vi "2_static_friction_main.vi"() -> ()   [LabVIEW 2019]
uses:
  helper_vis/TypeDef_Static_Friction.ctl
  helper_vis/TypeDef_Current_Setting.ctl
  Shared VIs/ENPID/PID_Settings.ctl
  Shared VIs/ENPID/Gains.ctl
  Shared VIs/ENPID/NonLinearGainParams.ctl
  Shared VIs/ENPID/NonLinearGain.ctl
  Shared VIs/ENPID/DPartVariable.ctl
  Shared VIs/ENPID/VelocityEstimate.ctl
  Shared VIs/ENPID/OutputRange.ctl
  Shared VIs/TypeDef_TDMS_States.ctl
  <vilib>/myRIO/Common/Instrument Driver Framework/myRIO v1.0/Encoder/typedefs/Encoder Signal Mode.ctl
  Shared VIs/ModelSpecific/ETHMikeModel.ctl
  Shared VIs/ModelSpecific/ReadOnlyGlobalActions.ctl
  <vilib>/myRIO/Instrument Drivers/Onboard IO/AI/typedefs/AI Reference.ctl
  <vilib>/myRIO/Common/Instrument Driver Framework/Utilities/typedefs/myRIO Generic Hardware Reference.ctl
  <vilib>/myRIO/Common/Instrument Driver Framework/Utilities/typedefs/Hardware Version Enum.ctl
  <vilib>/myRIO/Common/Instrument Driver Framework/Utilities/typedefs/myRIO v1.0 Reference.ctl
  <vilib>/myRIO/Common/Instrument Driver Framework/Utilities/typedefs/Generic FPGA Reference.ctl
  <vilib>/myRIO/Common/Instrument Driver Framework/myRIO v1.0/AI/typedefs/AI Channels List.ctl
  <vilib>/myRIO/Common/Instrument Driver Framework/myRIO v1.0/AI/typedefs/AI Channels Enum.ctl
  <vilib>/myRIO/Common/Instrument Driver Framework/Utilities/typedefs/Analog Scaling Constants List.ctl
  <vilib>/myRIO/Common/Instrument Driver Framework/Utilities/typedefs/Analog Scaling Constants.ctl
  <vilib>/userDefined/High Color/nirio_resource_hc.ctl
  <vilib>/myRIO/Instrument Drivers/Onboard IO/AO/typedefs/AO Reference.ctl
  <vilib>/myRIO/Common/Instrument Driver Framework/myRIO v1.0/AO/typedefs/AO Channels List.ctl
  <vilib>/myRIO/Common/Instrument Driver Framework/myRIO v1.0/AO/typedefs/AO Channels Enum.ctl
  <vilib>/Platform/TimedLoop/XDataNode/timing_clust.ctl
  <vilib>/Platform/TimedLoop/XDataNode/nitl_modes.ctl
  <vilib>/Platform/TimedLoop/XDataNode/wakeup.ctl
  <vilib>/Analysis/3filter.llb/Filter Passband Type.ctl
  <vilib>/myRIO/Common/Instrument Driver Framework/myRIO v1.0/AI/vis/myRIO v1.1 Open AI.vi
  <vilib>/myRIO/Common/Instrument Driver Framework/myRIO v1.0/AO/vis/myRIO v1.1 Open AO.vi
  <vilib>/myRIO/Common/Instrument Driver Framework/Utilities/vis/Validate Channels.vi
  <vilib>/myRIO/Common/Instrument Driver Framework/myRIO v1.0/AI/vis/myRIO v1.0 Reserve AI.vi
  <vilib>/myRIO/Common/Instrument Driver Framework/myRIO v1.0/AO/vis/myRIO v1.0 Reserve AO.vi
  <vilib>/myRIO/Common/Instrument Driver Framework/myRIO v1.0/AI/vis/myRIO v1.0 Close AI.vi
  <vilib>/myRIO/Common/Instrument Driver Framework/myRIO v1.0/Encoder/vis/myRIO v1.0 Close Encoder.vi
  <vilib>/myRIO/Common/Instrument Driver Framework/myRIO v1.0/AO/vis/myRIO v1.0 Close AO.vi
  <vilib>/myRIO/Common/Instrument Driver Framework/myRIO v1.0/AI/vis/myRIO v1.0 Build MUX Configuration AI.vi
  <vilib>/myRIO/Common/Instrument Driver Framework/myRIO v1.0/Resource Manager/vis/myRIO v1.0 Reserve Channel List.vi
  <vilib>/myRIO/Common/Instrument Driver Framework/myRIO v1.0/AO/vis/myRIO v1.0 Build MUX Configuration AO.vi
  <vilib>/myRIO/Common/Instrument Driver Framework/myRIO v1.0/AI/vis/myRIO v1.0 Unreserve AI.vi
  <vilib>/myRIO/Common/Instrument Driver Framework/myRIO v1.0/Encoder/vis/myRIO v1.0 Unreserve Encoder.vi
  <vilib>/myRIO/Common/Instrument Driver Framework/myRIO v1.0/AO/vis/myRIO v1.0 Unreserve AO.vi
  <vilib>/myRIO/Common/Instrument Driver Framework/myRIO v1.0/Resource Manager/vis/myRIO v1.0 Reserve Channel.vi
  <vilib>/myRIO/Common/Instrument Driver Framework/myRIO v1.0/Resource Manager/vis/myRIO v1.0 Unreserve Channel.vi
  <vilib>/myRIO/Common/Instrument Driver Framework/myRIO v1.0/Resource Manager/vis/myRIO v1.0 Unreserve Channel List.vi
  <vilib>/myRIO/Common/Instrument Driver Framework/myRIO v1.0/Encoder/vis/myRIO v1.0 Build MUX Configuration Encoder.vi
  <vilib>/myRIO/Common/Instrument Driver Framework/myRIO v1.0/Resource Manager/vis/myRIO v1.0 Build Mutex Name.vi
  <vilib>/myRIO/Common/Instrument Driver Framework/myRIO v1.0/Resource Manager/vis/myRIO v1.0 Create Configuration List.vi
  <vilib>/Utility/VariantDataType/GetNumericInfo.vi
  <vilib>/Utility/error.llb/Error Cluster From Error Code.vi
  <vilib>/myRIO/Common/Instrument Driver Framework/myRIO v1.0/myRIO v1.1 Open.vi
  <vilib>/myRIO/Common/Instrument Driver Framework/myRIO v1.0/AO/vis/myRIO v1.0 Get Scaling Constants AO.vi
  <vilib>/myRIO/Common/Instrument Driver Framework/Utilities/vis/IO Manager.vi
  <vilib>/myRIO/Common/Instrument Driver Framework/Utilities/vis/Configuration Manager.vi
  <vilib>/myRIO/Common/Instrument Driver Framework/myRIO v1.0/myRIO v1.0 Close.vi
  <vilib>/myRIO/Common/Instrument Driver Framework/myRIO v1.0/AO/vis/myRIO v1.0 Write AO.vi
  <vilib>/myRIO/Common/Instrument Driver Framework/myRIO v1.0/AI/vis/myRIO v1.0 Get Scaling Constants AI.vi
  <vilib>/myRIO/Common/Instrument Driver Framework/myRIO v1.0/Encoder/vis/myRIO v1.0 Read Encoder.vi
  <vilib>/myRIO/Common/Instrument Driver Framework/myRIO v1.0/AI/vis/myRIO v1.0 Read AI.vi
  <vilib>/myRIO/Common/Instrument Driver Framework/myRIO v1.0/Encoder/vis/myRIO v1.0 Enable Encoder.vi
  <vilib>/myRIO/Common/Instrument Driver Framework/myRIO v1.0/Encoder/vis/myRIO v1.0 Shutdown Encoder.vi
  <vilib>/myRIO/Common/Instrument Driver Framework/myRIO v1.0/Resource Manager/vis/myRIO v1.0 Configure IO.vi
  <vilib>/myRIO/Instrument Drivers/Onboard IO/AO/vis/myRIO AO Open.xnode
  <vilib>/myRIO/Instrument Drivers/Onboard IO/AI/vis/myRIO AI Open.xnode
  <vilib>/Platform/TimedLoop/XDataNode/XDataNode.xnode
  <vilib>/myRIO/Instrument Drivers/Onboard IO/AO/AO.lvlib
  <vilib>/myRIO/Instrument Drivers/Onboard IO/Encoder/Encoder.lvlib
  <vilib>/myRIO/Instrument Drivers/Onboard IO/AI/AI.lvlib
  <vilib>/addons/control/pid/NI_PID_pid.lvlib
  <vilib>/Analysis/NI_AALBase.lvlib
  <vilib>/ptbypt/NI_PtbyPt.lvlib
  <vilib>/Platform/TimedLoop/XDataNode/XDNodeRunTimeDep.lvlib
panel:
  in  "TDMS Storage File Input":string
  out "TDMS States":T1
  in  "PID Settings":T2={"Gains"={"K(e)"=0.0, "Kp"=0.800000011920929, "Ki"=0.0, "Kd"=0.003000000026077032}, "Non-linear gain"={"Non-linear gain P"=enum."off", "Non-linear gain I"=enum."off", "Non-linear gain D"=enum."off"}, "D-Part variable"=enum."process variable", "Velocity estimate dy/dt"=enum."external", "Anti reset windup"=TRUE, "I-Part error band"=inf, "Output range"={"output high"=0.0, "output low"=0.0}}
  in  "Save data?":bool
  out "Final Current Setpoint":dbl
  out "Boolean: Apply Current":bool
  out "Boolean: Move":bool
  out "Position Difference [deg]":dbl
  in  "move":bool
  out "Profile Complete?":bool
  in  "Current Direction [+/-]":T9
  out "Velocity [deg/s]":dbl
  in  "Actions":T10
  out "Current Setpoint [A]":dbl
  out "Position [deg] Chart":dbl(graph)
  out "Current [A] Chart":dbl(graph)
  out "Position [deg]":dbl
  in  "stop":bool
  out "Current [A]":dbl
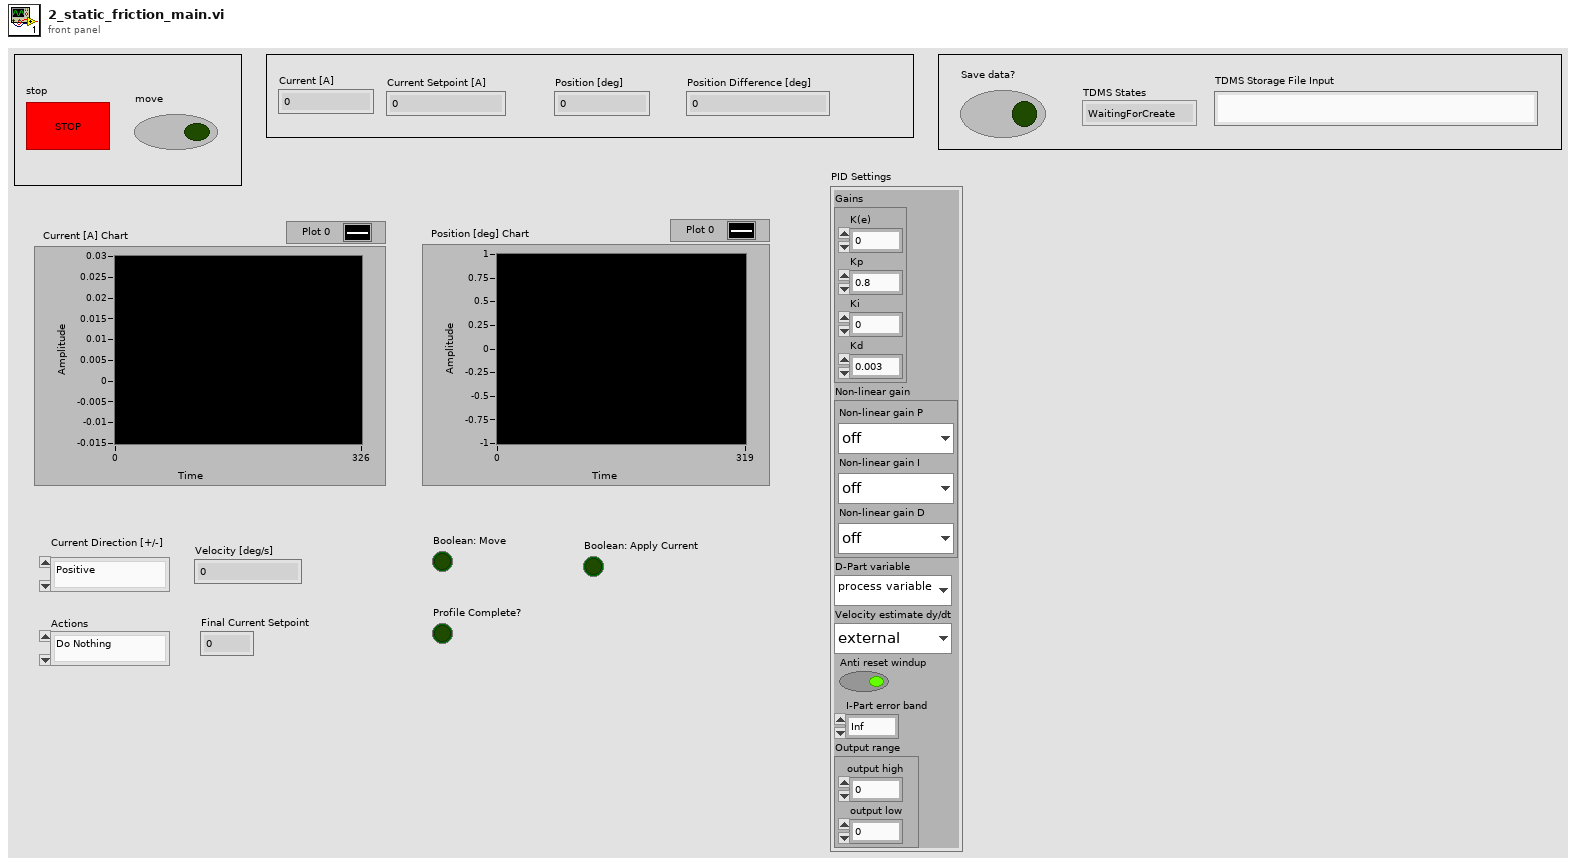
[diagram p1: front panel]
types:
  T1 = typedef "TypeDef_TDMS_States.ctl" = enum16{"WaitingForCreate", "Create", "Buffering", "Flushing", "Write", "Close"}
  T2 = typedef "PID_Settings.ctl" = cluster{"Gains":T3, "Non-linear gain":T4, "D-Part variable":T6, "Velocity estimate dy/dt":T7, "Anti reset windup":bool, "I-Part error band":dbl, "Output range":T8}
  T3 = typedef "Gains.ctl" = cluster{"K(e)":dbl, "Kp":dbl, "Ki":dbl, "Kd":dbl}
  T4 = typedef "NonLinearGainParams.ctl" = cluster{"Non-linear gain P":T5, "Non-linear gain I":T5, "Non-linear gain D":T5}
  T5 = typedef "NonLinearGain.ctl" = enum16{"exponential", "quadratic", "off"}
  T6 = typedef "DPartVariable.ctl" = enum16{"error", "process variable"}
  T7 = typedef "VelocityEstimate.ctl" = enum16{"derivative", "external"}
  T8 = typedef "OutputRange.ctl" = cluster{"output high":dbl, "output low":dbl}
  T9 = typedef "TypeDef_Current_Setting.ctl" = enum16{"Positive", "Negative"}
  T10 = typedef "TypeDef_Static_Friction.ctl" = enum16{"Do Nothing", "Move", "Wait", "Apply Current"}
  T11 = typedef "nirio_resource_hc.ctl" = tag
  T12 = typedef "Hardware Version Enum.ctl" = enum16{"Unknown", "myRIO-1900", "myRIO-1950", "roboRIO", "NI ELVIS RIO CM", "ELVIS III"}
  T13 = enum16{"open", "open or create", "create or replace", "create", "open (read-only)"}
  T14 = typedef "XDNodeRunTimeDep.lvlib/timing_clust.ctl" = cluster{"Expected End [f-1]":u64, "Actual End [f-1]":u64, "Finished Late? [f-1]":bool, "Expected End [i-1]":u64, "Actual End [i-1]":u64, "Finished Late? [i-1]":bool, "Expected Start [i]":u64, "Actual Start [i]":u64, "Expected Start [f]":u64, "Actual Start [f]":u64, "Source Name":string, "Structure Name":string, "Period":i64, "Deadline":i64, "Offset":i64, "Start":i64, "Priority":i32, "Timeout":i32, "Mode":T15, "Wakeup Reason":T16, "Error":errorcluster, "Source Type":string, "Secondary Source Type":string, "Global End Time":u64, "Global Start Time":u64, "Frame Duration":u64, "Iteration Duration":u64, "Assigned CPU":i32, "I/O Scan Engine Mode":u32}
  T15 = typedef "XDNodeRunTimeDep.lvlib/nitl_modes.ctl" = enum32{"No Change", "Process missed periods, maintain original phase", "Discard missed periods, maintain original phase", "Process missed periods, ignore original phase", "Discard missed periods, ignore original phase"}
  T16 = typedef "XDNodeRunTimeDep.lvlib/wakeup.ctl" = enum32{"Normal", "Aborted", "Asynchronous wakeup", "Timing source error", "Timed loop error", "Timeout"}
  T17 = typedef "NI_AALBase.lvlib/Filter Passband Type.ctl" = enum32{"Lowpass", "Highpass", "Bandpass", "Bandstop"}
  T18 = typedef "ReadOnlyGlobalActions.ctl" = enum16{"Initialize", "Read", "Write"}
  T19 = typedef "ETHMikeModel.ctl" = enum16{"ETH Mike #1", "ETH Mike #2", "ETH Mike #3", "ETH Mike #4", "ETH MIKE #5"}
  T20 = typedef "Encoder Signal Mode.ctl" = enum16{"Quadrature phase signal", "Step and direction signal"}
  T21 = typedef "AO.lvlib/AO Reference.ctl" = cluster{"myRIO Reference":T22, "AO Channel List":T25, "AO Scaling Constant List":T27}
  T22 = typedef "myRIO Generic Hardware Reference.ctl" = cluster{"myRIO Model":T12, "myRIO Hardware Reference":T23}
  T23 = typedef "myRIO v1.0 Reference.ctl" = cluster{"Generic FPGA Reference":T24, "Allow multiple opens":bool}
  T24 = typedef "Generic FPGA Reference.ctl" = refnum<k20>
  T25 = typedef "AO Channels List.ctl" = T26[]
  T26 = typedef "AO Channels Enum.ctl" = enum16{"Not Connected", "AudioOut/Left", "AudioOut/Right", "C/AO0", "C/AO1", "A/AO0", "A/AO1", "B/AO0", "B/AO1"}
  T27 = typedef "Analog Scaling Constants List.ctl" = T28[]
  T28 = typedef "Analog Scaling Constants.ctl" = cluster{"LSB Weight (Volts)":dbl, "Offset (Volts)":dbl, "Signed?":bool}
  T29 = typedef "Encoder.lvlib/Encoder Reference.ctl" = cluster{"myRIO Reference":T22, "Encoder Channels Enum":T30}
  T30 = typedef "Encoder Channels Enum.ctl" = enum16{"Not Connected", "C/ENC0", "C/ENC1", "A/ENC", "A/ENC0", "A/ENC1", "A/ENC2", "A/ENC3", "A/ENC4", "A/ENC5", "A/ENC6", "A/ENC7", "A/ENC8", "A/ENC9", "B/ENC", "B/ENC0", "B/ENC1", "B/ENC2", "B/ENC3", "B/ENC4", "B/ENC5", "B/ENC6", "B/ENC7", "B/ENC8", "B/ENC9", "DIO/ENC0", "DIO/ENC1", "DIO/ENC2", "DIO/ENC3", "DIO/ENC4"}
  T31 = typedef "AI.lvlib/AI Reference.ctl" = cluster{"myRIO Reference":T22, "AI Channels List":T32, "AI Scaling Constants List":T27}
  T32 = typedef "AI Channels List.ctl" = T33[]
  T33 = typedef "AI Channels Enum.ctl" = enum16{"Not Connected", "AudioIn/Left", "AudioIn/Right", "C/AI0", "C/AI1", "A/AI0", "A/AI1", "A/AI2", "A/AI3", "A/AI4", "A/AI5", "A/AI6", "A/AI7", "B/AI0", "B/AI1", "B/AI2", "B/AI3", "B/AI4", "B/AI5", "B/AI6", "B/AI7", "AI/AI0", "AI/AI1", "AI/AI2", "AI/AI3", "A/AI0 (DIFF)", "A/AI1 (DIFF)", "A/AI2 (DIFF)", "A/AI3 (DIFF)", "B/AI0 (DIFF)", "B/AI1 (DIFF)", "B/AI2 (DIFF)", "B/AI3 (DIFF)"}
  T34 = typedef "TypeDefTachometerParam.ctl" = cluster{"Offset [V]":dbl, "Gain [deg/sV]":dbl}
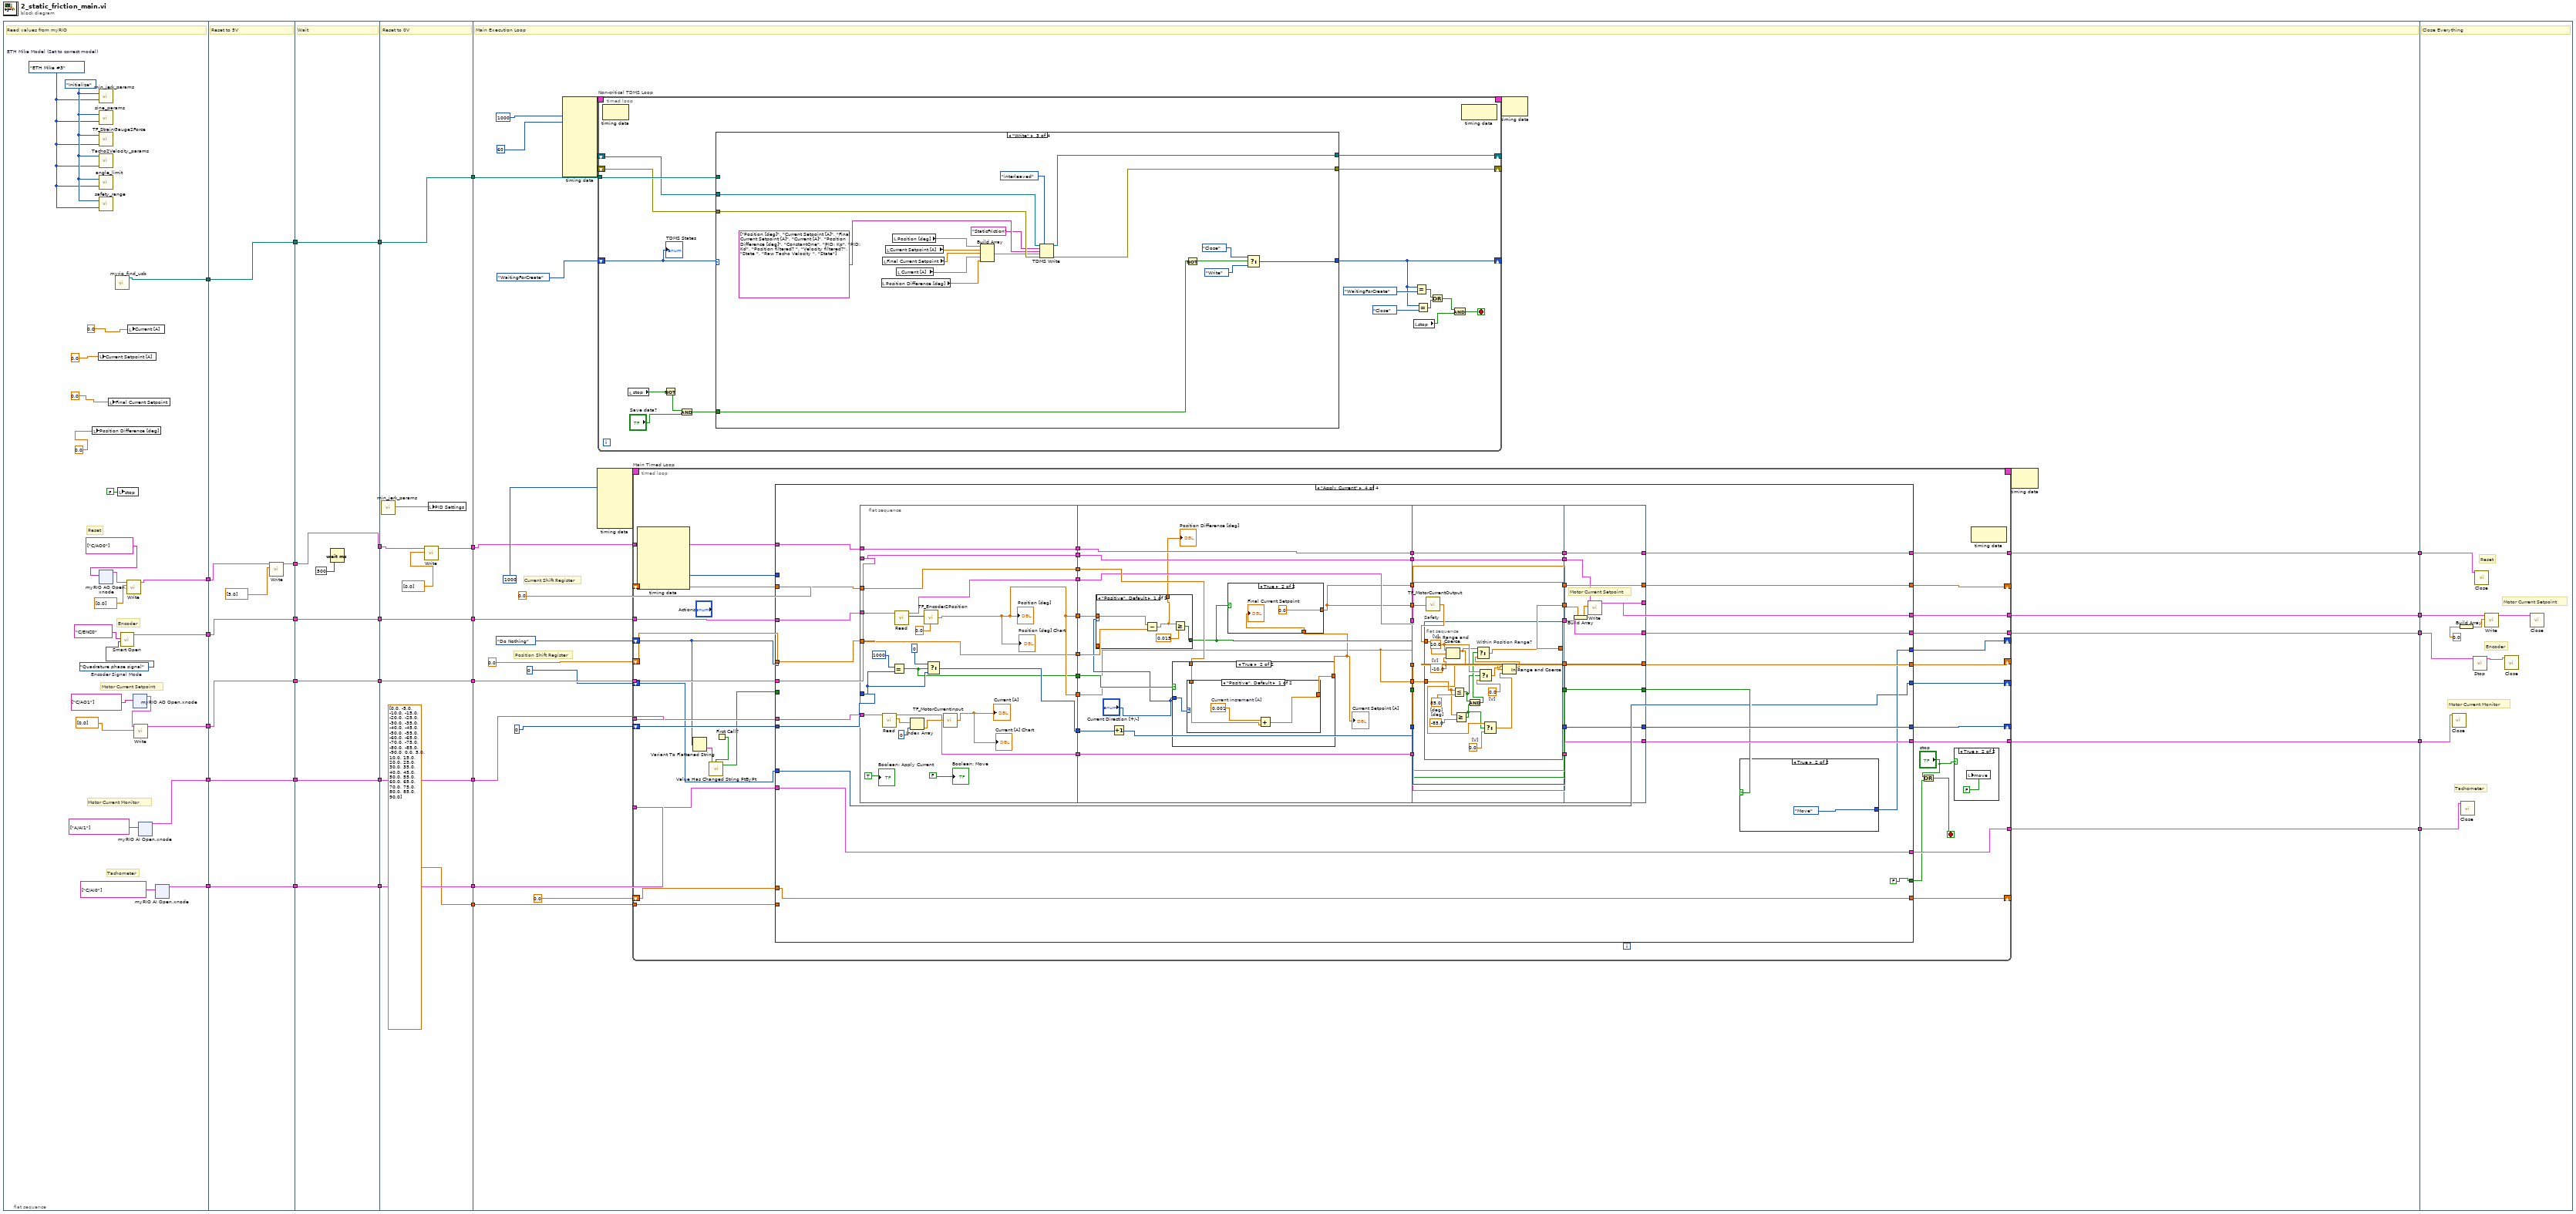
[diagram p0: block diagram]
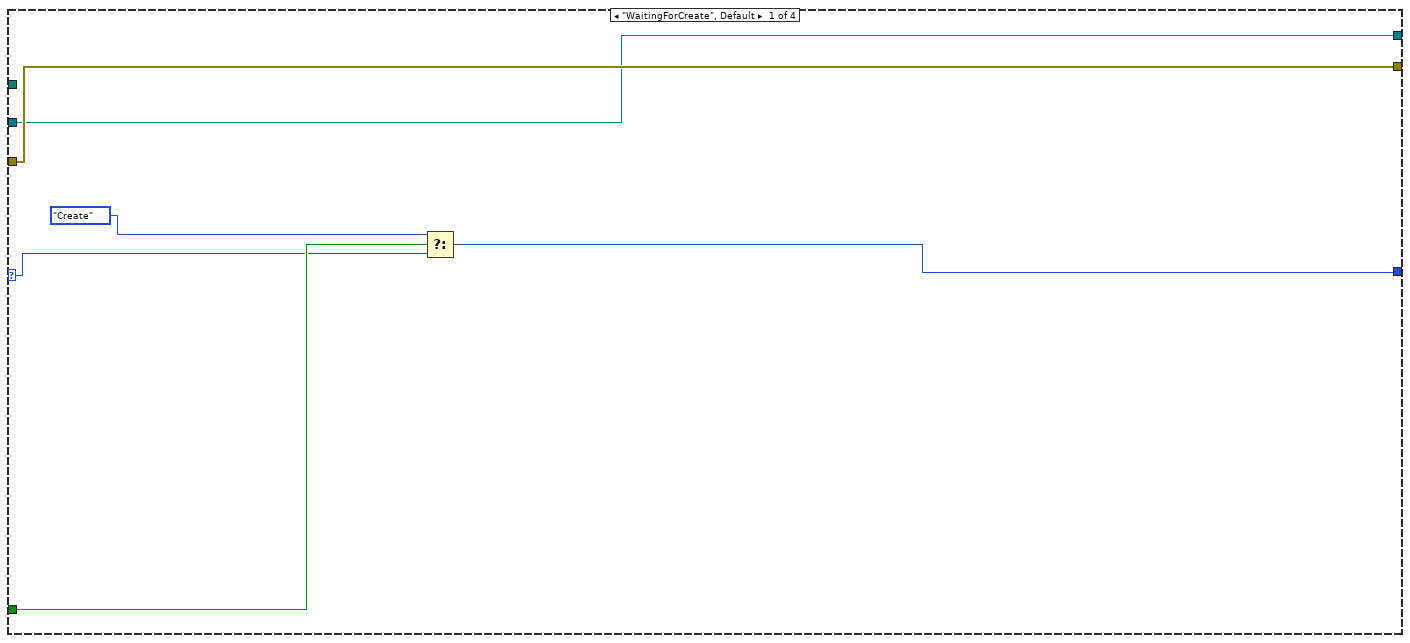
[diagram p2: hidden frame]
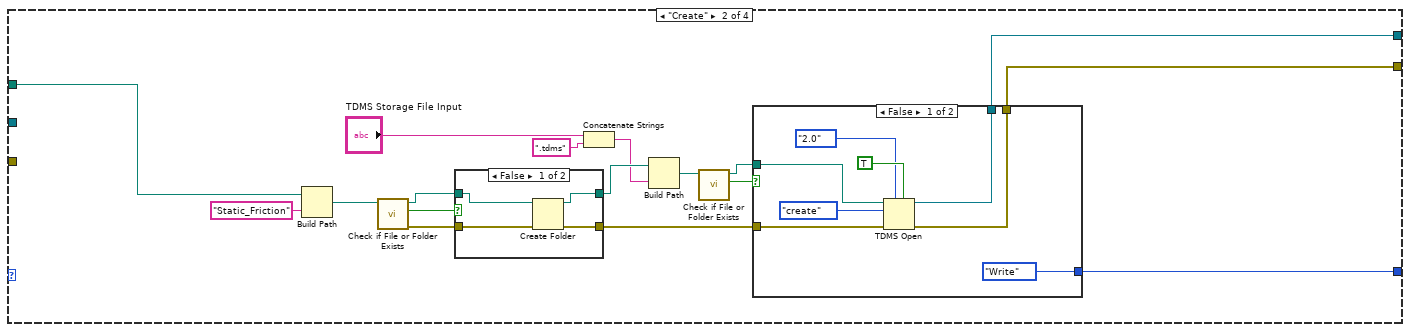
[diagram p3: hidden frame]
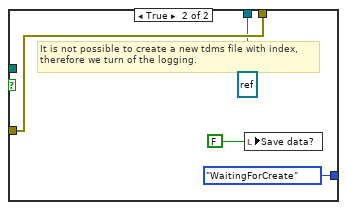
[diagram p4: hidden frame]
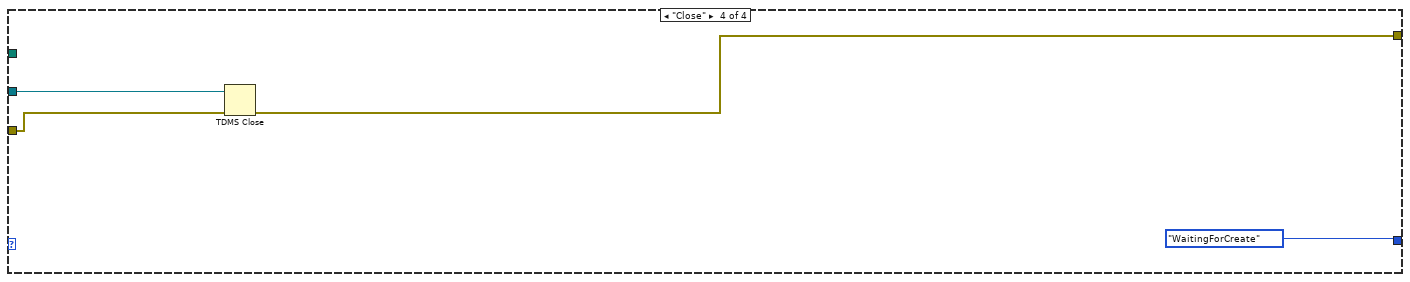
[diagram p6: hidden frame]
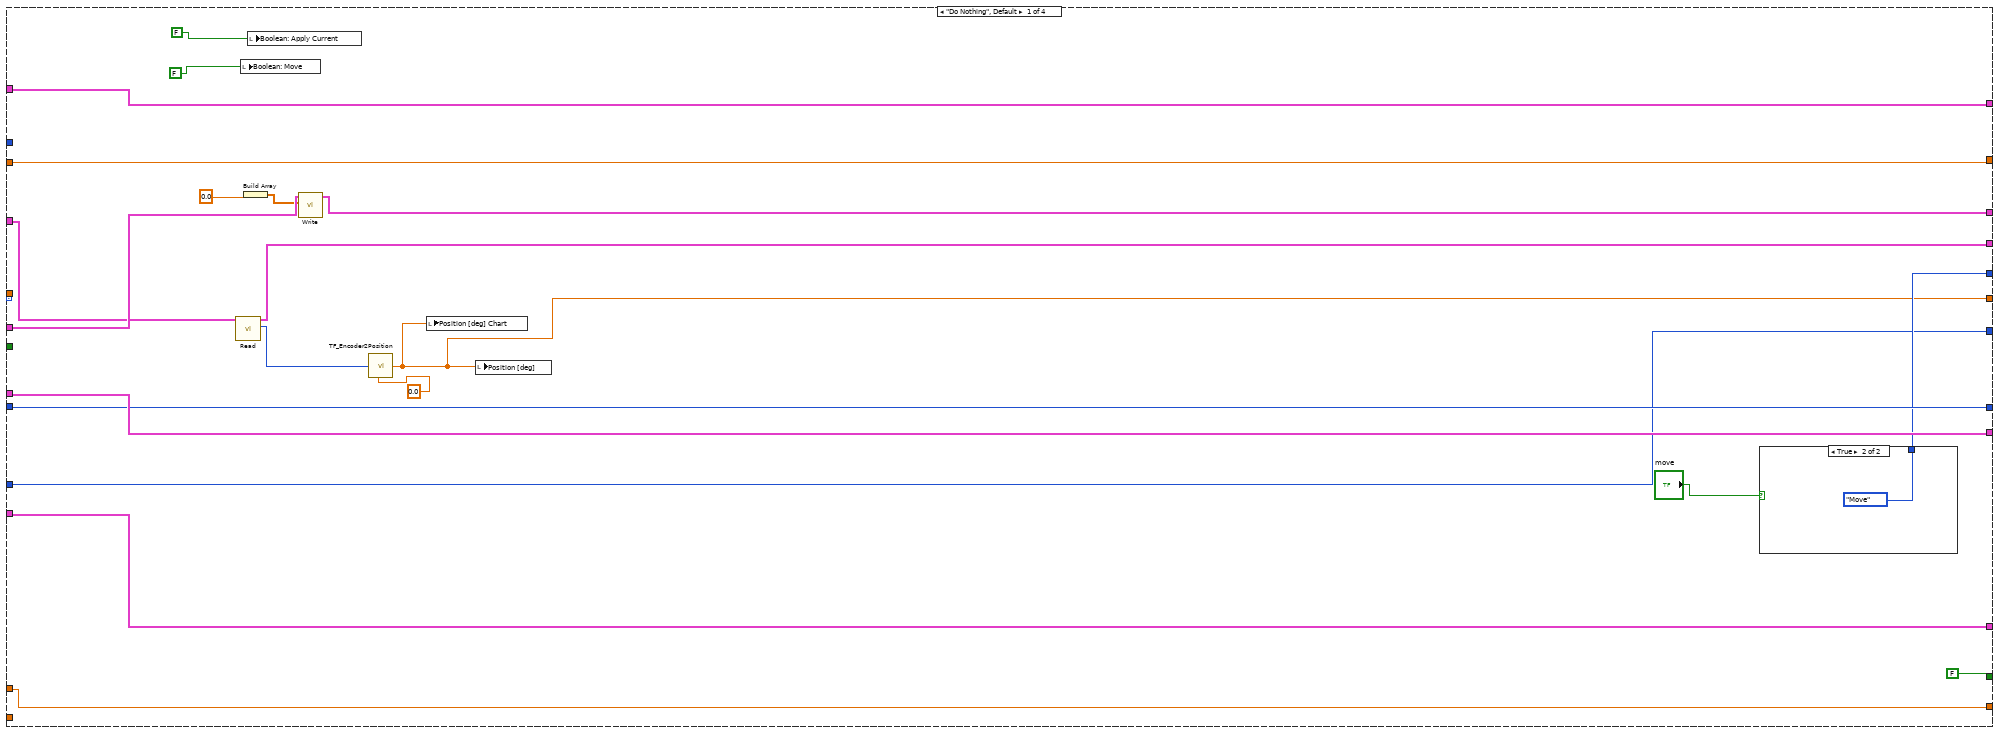
[diagram p8: hidden frame]
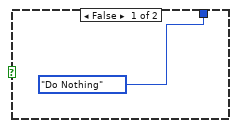
[diagram p9: hidden frame]
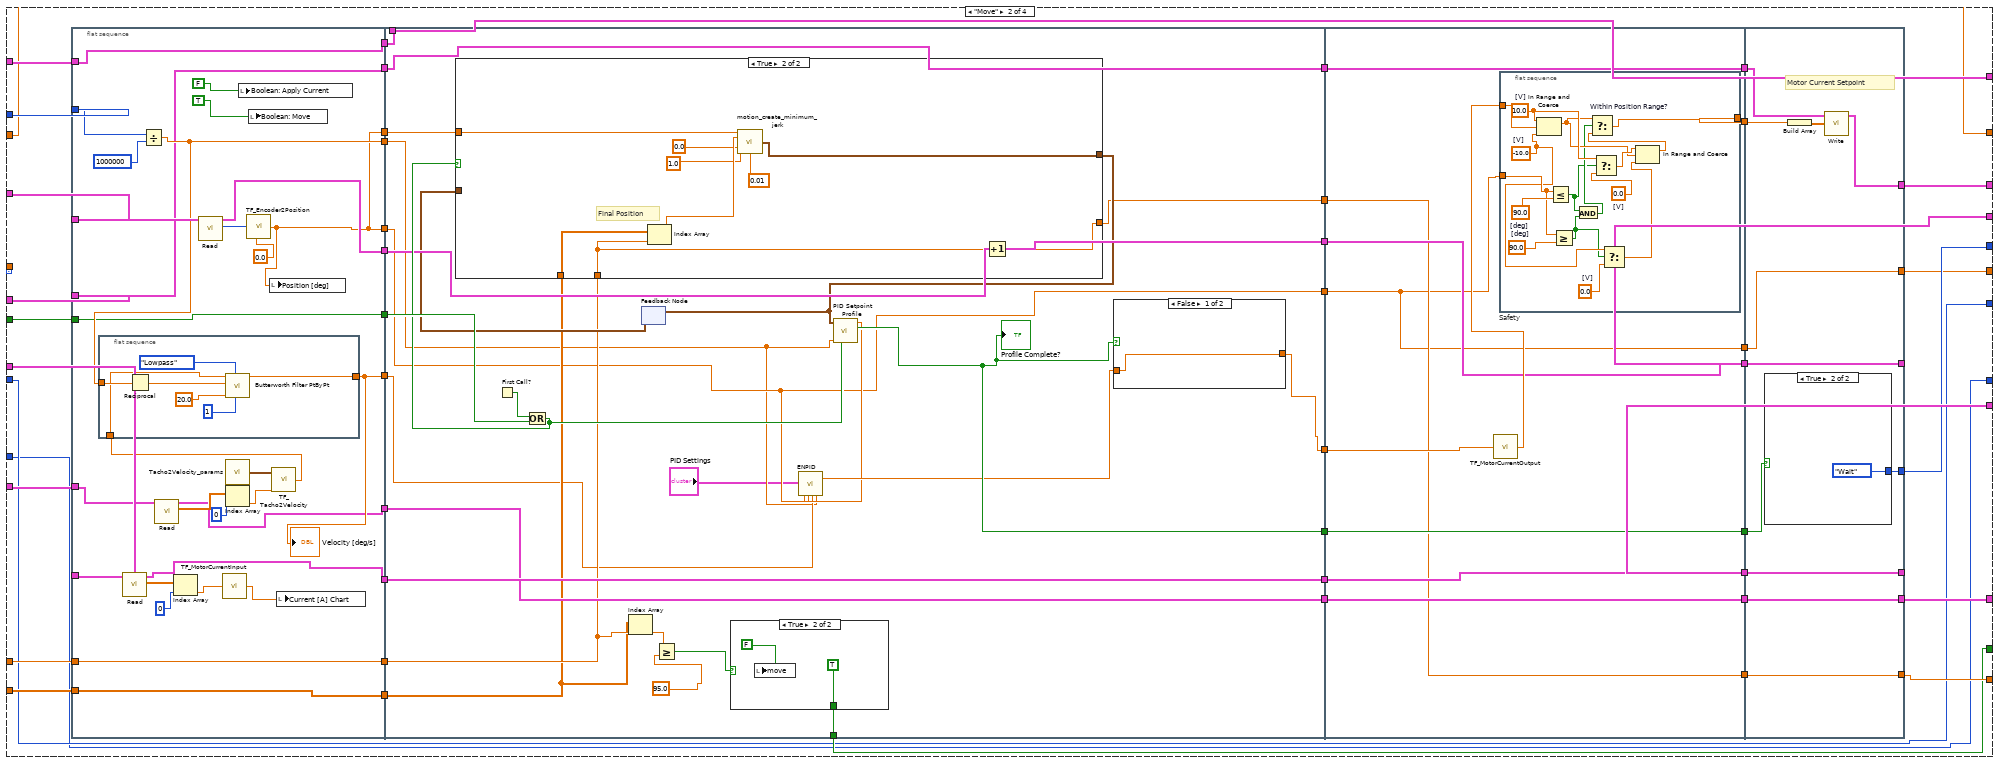
[diagram p10: hidden frame]
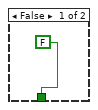
[diagram p11: hidden frame]
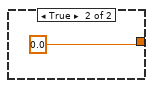
[diagram p12: hidden frame]
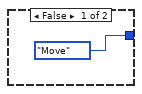
[diagram p14: hidden frame]
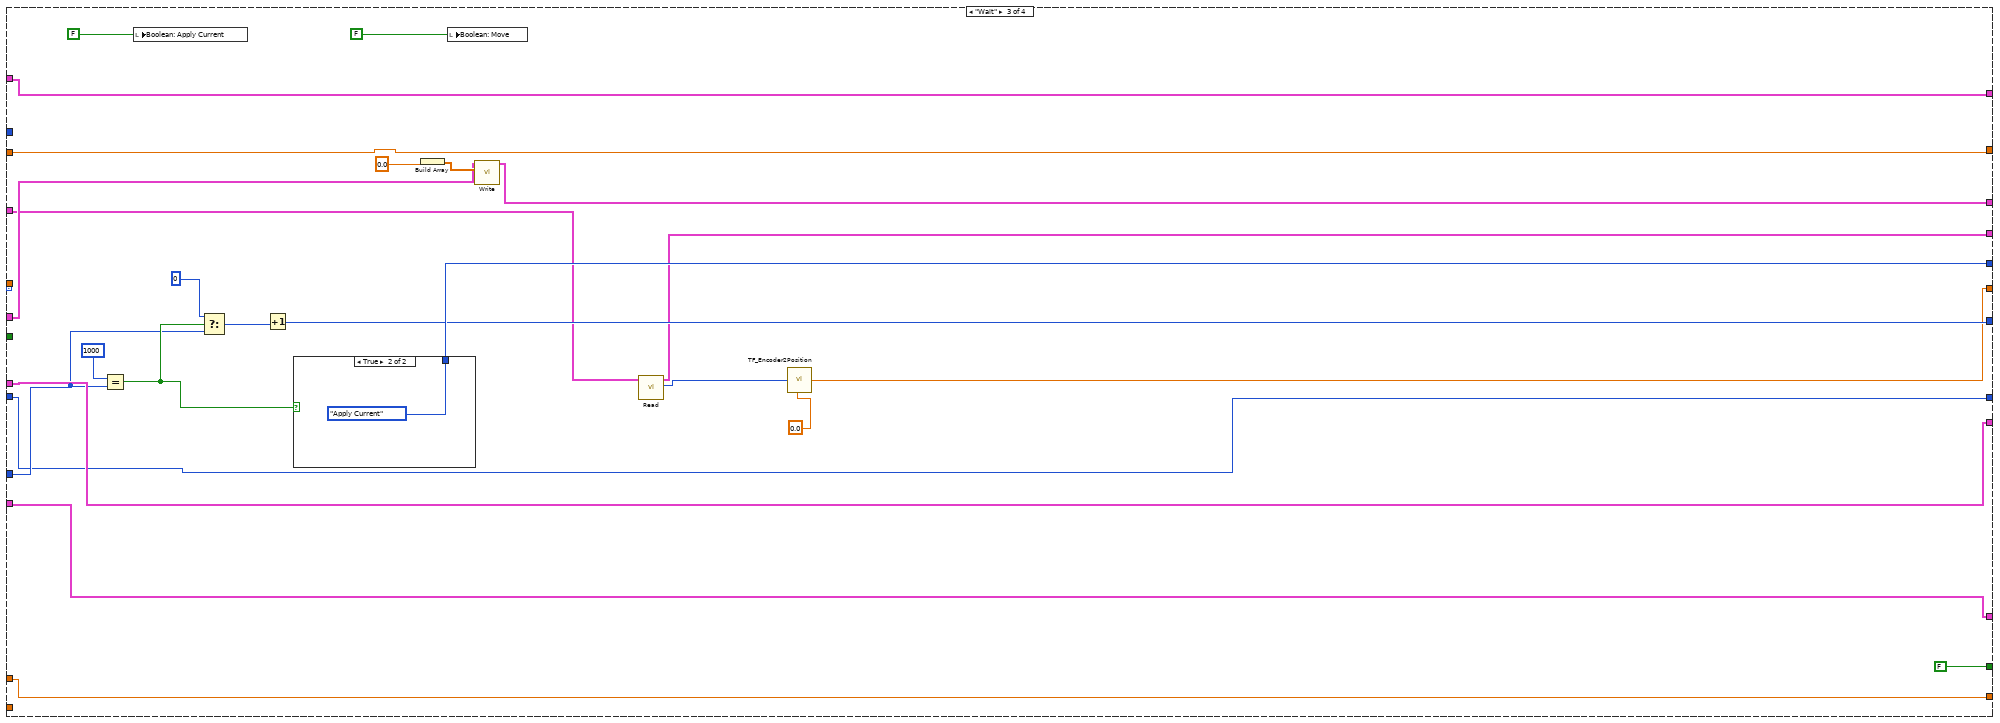
[diagram p15: hidden frame]
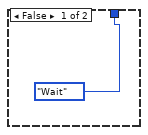
[diagram p16: hidden frame]
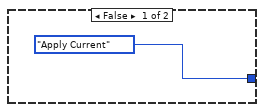
[diagram p17: hidden frame]
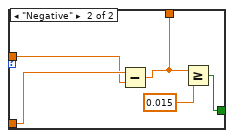
[diagram p18: hidden frame]
diagram:
  n1 = flat-sequence {
    tunnel: [w50] -> w30
    tunnel: [w47] -> w26
    tunnel: [w43] -> w25
    tunnel: [w41] -> w24
    tunnel: [w39] -> w7
    tunnel: [w38] -> w1
    tunnel: w30 -> [w132]
    tunnel: [w131] -> w28
    tunnel: w26 -> [w130]
    tunnel: w25 -> [w129]
    tunnel: w24 -> [w128]
    tunnel: [w130] -> w21
    tunnel: [w129] -> w18
    tunnel: [w128] -> w15
    tunnel: [w127] -> w8
    tunnel: w7 -> [w127]
    tunnel: [w126] -> w2
    tunnel: w1 -> [w126]
    tunnel: [w139] -> w29
    tunnel: w28 -> [w139]
    tunnel: [w138] -> w22
    tunnel: w21 -> [w138]
    tunnel: [w137] -> w19
    tunnel: w18 -> [w137]
    tunnel: [w136] -> w16
    tunnel: w15 -> [w136]
    tunnel: [w135] -> w9
    tunnel: w8 -> [w135]
    tunnel: [w134] -> w3
    tunnel: w2 -> [w134]
    tunnel: w29 -> [w149]
    tunnel: [w148] -> w27
    tunnel: [w147] -> w23
    tunnel: w22 -> [w147]
    tunnel: [w146] -> w20
    tunnel: w19 -> [w146]
    tunnel: [w145] -> w17
    tunnel: w16 -> [w145]
    tunnel: [w144] -> w10
    tunnel: w9 -> [w144]
    tunnel: [dbl[] [0.0, -5.0, -10.0, -15.0, -20.0, -25.0, -30.0, -35.0, -40.0, -45.0, -50.0, -55.0, -60.0, -65.0, -70.0, -75.0, -80.0, -85.0, -90.0, 0.0, 5.0, 10.0, 15.0, 20.0, 25.0, 30.0, 35.0, 40.0, 45.0, 50.0, 55.0, 60.0, 65.0, 70.0, 75.0, 80.0, 85.0, 90.0]] -> w5
    tunnel: [w142] -> w4
    tunnel: w3 -> [w142]
    tunnel: w27 -> [w169]
    tunnel: w23 -> [w173]
    tunnel: w20 -> [w172]
    tunnel: w17 -> [w163]
    tunnel: [w168] -> w14
    tunnel: [w167] -> w13
    tunnel: [w166] -> w12
    tunnel: [w165] -> w11
    tunnel: w10 -> [w164]
    tunnel: [w162] -> w6
    tunnel: w5 -> [w160]
    tunnel: w4 -> [w152]
    tunnel: w14 -> [w678]
    tunnel: w13 -> [w673]
    tunnel: w12 -> [w672]
    tunnel: w11 -> [w671]
    tunnel: w6 -> [w670]
    frame #0 {
      w33 = ReadOnlyGlobalActions."Initialize" ("Action (Read)")
      w32 = ETHMikeModel."ETH Mike #3"  # ETH Mike Model (Set to correct model)
      w48 = Encoder_Signal_Mode."Quadrature phase signal"  # Encoder Signal Mode
      # "Tachometer"
      # "Motor Current Monitor"
      # "Motor Current Setpoint"
      # "Encoder"
      # "Reset"
      # "Read values from myRIO"
      n2 = local write "Position Difference [deg]"(0.0) -> ()
      n3 = local write "Current Setpoint [A]"(0.0) -> ()
      n4 = call "min_jerk_params.vi"("Action (Read)"=w33, "ETH Mike Model"=w32) -> ()  [unwired: 17 in, 1 out]
      n5 = call "sine_params.vi"("Action (Read)"=w33, "ETH Mike Model"=w32) -> ()  [unwired: 17 in, 1 out]
      n6 = call "TF_StrainGauge2Force.vi"("Action (Read)"=w33, "ETH Mike Model"=w32) -> ()  [unwired: 3 in, 1 out]
      n7 = call "Tacho2Velocity_params.vi"("Action (Read)"=w33, "ETH Mike Model"=w32) -> ()  [unwired: 3 in, 1 out]
      n8 = call "angle_limit.vi"("ETH Mike Model"=w32, "Action (Read)"=w33) -> ()  [unwired: 1 out]
      n9 = call "safety_range.vi"("ETH Mike Model"=w32, "Action (Read)"=w33) -> ()  [unwired: 1 out]
      n10 = xnode "myRIO AO Open.xnode"("Channel Names"=tag[] ["C/AO0"]) -> ("AO Ref Out"=w52:T21)  [unwired: 2 in, 1 out]
      n11 = local write "Final Current Setpoint"(0.0) -> ()
      n12 = call "myrio_find_usb.vi"() -> ("Largest USB Partition Path"=w38:path)  [unwired: 9 in, 2 out]
      n13 = local write "stop"(FALSE ("stop")) -> ()
      n14 = call <vilib>:"Smart Open.vi"("Encoder Signal Mode"=w48, "Channel Name"=tag "C/ENC0") -> ("Encoder Ref Out"=w47:T29)  [unwired: 8 in, 1 out]
      n15 = call <vilib>:"Write.vi"("Values"=dbl[] [0.0], "AO Ref In"=w52) -> ("AO Ref Out"=w50:T21)  [unwired: 7 in, 1 out]
      n16 = local write "Current [A]"(0.0) -> ()
      n17 = xnode "myRIO AO Open.xnode"("Channel Names"=tag[] ["C/AO1"]) -> ("AO Ref Out"=w45:T21)  [unwired: 2 in, 1 out]
      n18 = call <vilib>:"Write.vi"("Values"=dbl[] [0.0], "AO Ref In"=w45) -> ("AO Ref Out"=w43:T21)  [unwired: 7 in, 1 out]
      n19 = xnode "myRIO AI Open.xnode"("Channel Names"=tag[] ["A/AI1"]) -> ("AI Ref Out"=w41:T31)  [unwired: 2 in, 1 out]
      n20 = xnode "myRIO AI Open.xnode"("Channel Names"=tag[] ["C/AI0"]) -> ("AI Ref Out"=w39:T31)  [unwired: 2 in, 1 out]
    }
    frame #1 {
      # "Reset to 5V"
      n21 = call <vilib>:"Write.vi"("Values"=dbl[] [5.0], "AO Ref In"=w132) -> ("AO Ref Out"=w131:T21)  [unwired: 7 in, 1 out]
    }
    frame #2 {
      # "Wait"
      n22 = Wait (ms)(milliseconds to wait=500) -> ()  [unwired: 1 out]
    }
    frame #3 {
      # "Reset to 0V"
      n23 = call "min_jerk_params.vi"() -> ("PID Settings"=w141:T2)  [unwired: 19 in]
      n24 = call <vilib>:"Write.vi"("Values"=dbl[] [0.0], "AO Ref In"=w149) -> ("AO Ref Out"=w148:T21)  [unwired: 7 in, 1 out]
      n25 = local write "PID Settings"(w141) -> ()
    }
    frame #4 {
      # "Position Shift Register"
      # "Current Shift Register"
      # "Main Execution Loop"
      n26 = node-c288(1000, 60) -> (w156:T14)  [unwired: 8 in]
      n27 = node-c288(1000) -> (w176:T14)  [unwired: 6 in]
      n28 = timed-loop "Non-critical TDMS Loop" {
        timing: w156 -> [_]
        timing-out: [_] -> w155
        tunnel: w152 -> [w194]
        shift-right: [w183] -> _
        shift-left: TypeDef_TDMS_States."WaitingForCreate" ("TDMS States") -> [w189]
        shift-right: [w193] -> _
        shift-left: _ -> [w190]
        shift-right: [w192] -> _
        shift-left: _ -> [w191]
        stop <- w177 stop-if-true
        n29 = node-c288() -> ()  [unwired: 1 in, 1 out]
        n30 = local read "stop"() -> (w188:bool)
        n31 = Not(x=w188) -> (.not. x?=w186:bool)
        n32 = And(x=w186, y="Save data?") -> (x .and. y?=w185:bool)
        n33 = case shown="\"Write\"" w189 {
          selector: w189 -> [w198 _ _ _]
          tunnel: w185 -> [w199 _ w240 _]
          tunnel: [w197 w201 w236 TypeDef_TDMS_States."WaitingForCreate" ("TDMS States")] -> w183
          tunnel: w194 -> [_ w204 _ _]
          tunnel: [w195 w202 w242 _] -> w193
          tunnel: [w196 w203 w241 w254] -> w192
          tunnel: w191 -> [w196 _ w248 w256]
          tunnel: w190 -> [w195 _ w245 w255]
          frame "WaitingForCreate", Default {
            n34 = Select(t=TypeDef_TDMS_States."Create" ("TDMS States"), s=w199, f=w198) -> (s? t:f=w197:T1)
          }
          frame "Create" {
            n35 = Build Path(base path=w204, name or relative path="Static_Friction") -> (appended path=w206:path)
            n36 = call <vilib>:"Check if File or Folder Exists.vi"("path"=w206) -> ("error out"=w215:errorcluster, "file or folder exists?"=w217:bool, "dup path"=w216:path)  [unwired: 8 in]
            n37 = case shown="False" w217 {
              tunnel: w216 -> [w233 w234]
              tunnel: [w232 w235] -> w210
              tunnel: w215 -> [w231 w235]
              tunnel: [w230 w234] -> w214
              frame False {
                n38 = Create Folder(path (use dialog)=w233, error in=w231) -> (created path=w230:path, error out=w232:errorcluster)  [unwired: 1 in, 1 out]
              }
              frame True {
              }
            }
            n39 = Concatenate Strings("TDMS Storage File Input", ".tdms") -> (w211:string)
            n40 = Build Path(base path=w214, name or relative path=w211) -> (appended path=w209:path)
            n41 = call <vilib>:"Check if File or Folder Exists.vi"("path"=w209) -> ("file or folder exists?"=w208:bool, "dup path"=w207:path)  [unwired: 8 in, 1 out]
            n42 = case shown="False" w208 {
              tunnel: [TypeDef_TDMS_States."Write" ("TDMS States") TypeDef_TDMS_States."WaitingForCreate" ("TDMS States")] -> w201
              tunnel: [w224 refnum<k34> refnum ("tdms file out")] -> w202
              tunnel: [w223 w228] -> w203
              tunnel: w210 -> [w219 w228]
              tunnel: w207 -> [w218 _]
              frame False {
                n43 = TDMS Open(5:TRUE, 7:enum16{"1.0", "2.0"}."2.0" ("file format version (2.0)"), 8:w219, 10:T13."create" ("operation (0:open)"), 11:w218) -> (0:w223:errorcluster, 3:w224:refnum<k34>)  [unwired: 2 in]
              }
              frame True {
                # "It is not possible to create a new tdms file with index,\ntherefore we turn of the logging."
                n44 = local write "Save data?"(FALSE ("Save data?")) -> ()
              }
            }
          }
          frame "Write" {
            n45 = local read "Position Difference [deg]"() -> (w253:dbl)
            n46 = local read "Final Current Setpoint"() -> (w251:dbl)
            n47 = local read "Current Setpoint [A]"() -> (w250:dbl)
            n48 = local read "Position [deg]"() -> (w249:dbl)
            n49 = local read "Current [A]"() -> (w252:dbl)
            n50 = Build Array(w249, w250, w251, w252, w253) -> (w247:dbl[])
            n51 = TDMS Write(0:w245, 1:enum16{"decimated", "interleaved"}."interleaved" ("data layout (0:decimated)"), 5:"StaticFriction" ("group name in (Untitled)"), 7:string[] ["Position [deg]", "Current Setpoint [A]", "Final Current Setpoint [A]", "Current [A]", "Position Difference [deg]", "ConstantOne", "PID: Kp", "PID: Kd", "Position filtered? ", "Velocity filtered?", "State ", "Raw Tacho Velocity ", "State"], 9:w247, 11:w248) -> (4:w242:refnum<k34>, 15:w241:errorcluster)  [unwired: 2 out]
            n52 = Not(x=w240) -> (.not. x?=w239:bool)
            n53 = Select(t=TypeDef_TDMS_States."Close" ("TDMS States"), s=w239, f=TypeDef_TDMS_States."Write" ("TDMS States")) -> (s? t:f=w236:T1)
          }
          frame "Close" {
            n54 = TDMS Close(8:w256, 11:w255) -> (0:w254:errorcluster)  [unwired: 1 out]
          }
        }
        n55 = local read "stop"() -> (w178:bool)
        n56 = Equal?(x=w183, y=TypeDef_TDMS_States."WaitingForCreate" ("TDMS States")) -> (x = y?=w181:bool)
        n57 = Equal?(x=w183, y=TypeDef_TDMS_States."Close" ("TDMS States")) -> (x = y?=w180:bool)
        n58 = Or(x=w181, y=w180) -> (x .or. y?=w179:bool)
        n59 = And(x=w179, y=w178) -> (x .and. y?=w177:bool)
        n60 = node-c288() -> ()  [unwired: 1 in, 1 out]
        "TDMS States" <- w189
      }
      n61 = timed-loop "Main Timed Loop" {
        timing: w176 -> [_]
        timing-out: [_] -> w175
        tunnel: w173 -> [w293]
        tunnel: w172 -> [w286]
        tunnel: w163 -> [w294]
        shift-right: [w292] -> _
        shift-left: 0.0 -> [w291]
        shift-right: [w290] -> _
        shift-left: 0 -> [w289]
        shift-right: [w288] -> _
        shift-left: 0.0 -> [w287]
        tunnel: w169 -> [w285]
        tunnel: [w284] -> w168
        tunnel: [w283] -> w167
        tunnel: [w279] -> w166
        tunnel: [w282] -> w165
        tunnel: w164 -> [w280]
        tunnel: [w278] -> w162
        shift-right: [w275] -> _
        shift-left: TypeDef_Static_Friction."Do Nothing" ("Actions") -> [w274]
        tunnel: w160 -> [w272]
        shift-right: [w271] -> _
        shift-left: 0.0 -> [w270]
        shift-right: [w267] -> _
        shift-left: 0 -> [w266]
        stop <- w269 stop-if-true
        n62 = node-c288() -> (w281:i64)  [unwired: 1 in, 7 out]
        n63 = Variant To Flattened String(Variant=w274) -> (data string=w277:string)  [unwired: 1 out]
        n64 = First Call?() -> (First Call?: T/F=w276:bool)
        n65 = call "Value Has Changed String PtByPt.vi"("input data point"=w277, "initialize"=w276) -> ("has changed"=w273:bool)  [unwired: 1 out]
        n66 = case shown="\"Apply Current\"" w274 {
          tunnel: w294 -> [w314 w364 w498 w531]
          tunnel: w293 -> [w303 w366 w488 w530]
          tunnel: [w315 w323 w499 w529] -> w292
          tunnel: w291 -> [w315 w323 w499 w528]
          tunnel: [w313 w321 w493 w527] -> w290
          tunnel: w289 -> [w313 w322 w493 w526]
          tunnel: [w296 w320 w485 w525] -> w288
          tunnel: w287 -> [_ _ _ w524]
          tunnel: w286 -> [w310 w363 w504 w523]
          tunnel: w285 -> [w316 w361 w507 w522]
          tunnel: [w316 w360 w507 w521] -> w284
          tunnel: [w308 w362 w503 w520] -> w283
          tunnel: [w302 w359 w489 w519] -> w279
          tunnel: [w314 w358 w498 w518] -> w282
          tunnel: w281 -> [_ w367 _ _]
          tunnel: w280 -> [w312 w365 w497 w517]
          tunnel: [w312 w357 w497 w517] -> w278
          tunnel: [w306 w333 w505 w515] -> w275
          tunnel: w273 -> [_ w334 _ _]
          tunnel: w272 -> [_ w331 _ _]
          tunnel: [w304 w327 w495 w513] -> w271
          tunnel: w270 -> [w304 w326 w495 w513]
          tunnel: [FALSE w325 FALSE FALSE] -> w268
          tunnel: w266 -> [w299 w321 w494 w512]
          tunnel: [w299 w322 w492 w512] -> w267
          frame "Do Nothing", Default {
            n67 = call <vilib>:"Read.vi"("Encoder Ref In"=w303) -> ("Counter Value"=w301:i32, "Encoder Ref Out"=w302:T29)  [unwired: 6 in, 3 out]
            n68 = local write "Boolean: Move"(FALSE) -> ()
            n69 = Build Array(0.0) -> (w309:dbl[])
            n70 = local write "Boolean: Apply Current"(FALSE) -> ()
            n71 = call <vilib>:"Write.vi"("Values"=w309, "AO Ref In"=w310) -> ("AO Ref Out"=w308:T21)  [unwired: 7 in, 1 out]
            n72 = call "TF_Encoder2Position.vi"("Counter Value"=w301, "Offset"=0.0) -> ("Position [deg]"=w296:dbl)  [unwired: 3 in]
            n73 = local write "Position [deg] Chart"(w296) -> ()
            n74 = local write "Position [deg]"(w296) -> ()
            n75 = case shown="True" "move" {
              tunnel: [TypeDef_Static_Friction."Do Nothing" ("Actions") TypeDef_Static_Friction."Move" ("Actions")] -> w306
              frame False {
              }
              frame True {
              }
            }
          }
          frame "Move" {
            n76 = flat-sequence {
              tunnel: w367 -> [w389]
              tunnel: w366 -> [w395]
              tunnel: [w373] -> w356
              tunnel: w365 -> [w392]
              tunnel: [w388] -> w355
              tunnel: [w387] -> w354
              tunnel: w364 -> [w382]
              tunnel: w363 -> [w381]
              tunnel: [w381] -> w353
              tunnel: w334 -> [w380]
              tunnel: [w380] -> w352
              tunnel: [w379] -> w351
              tunnel: w361 -> [w379]
              tunnel: [w378] -> w350
              tunnel: [w377] -> w349
              tunnel: [w376] -> w348
              tunnel: [w375] -> w332
              tunnel: w326 -> [w375]
              tunnel: w331 -> [w374]
              tunnel: [w374] -> w330
              tunnel: [w373] -> w324
              tunnel: w356 -> [w407]
              tunnel: w355 -> [w405]
              tunnel: w354 -> [w406]
              tunnel: w353 -> [w425]
              tunnel: [w418] -> w347
              tunnel: w352 -> [w428]
              tunnel: [w407] -> w346
              tunnel: w351 -> [w426]
              tunnel: [w426] -> w360
              tunnel: [w425] -> w345
              tunnel: [w424] -> w344
              tunnel: w350 -> [w424]
              tunnel: w349 -> [w423]
              tunnel: [w423] -> w343
              tunnel: w348 -> [w422]
              tunnel: [w422] -> w342
              tunnel: [w419] -> w341
              tunnel: w332 -> [w413]
              tunnel: w330 -> [w412]
              tunnel: [w417] -> w329
              tunnel: [w415] -> w325
              tunnel: w324 -> [w414]
              tunnel: w347 -> [w455]
              tunnel: w346 -> [w446]
              tunnel: [w453] -> w340
              tunnel: [w452] -> w339
              tunnel: w345 -> [w452]
              tunnel: w344 -> [w451]
              tunnel: [w451] -> w338
              tunnel: w343 -> [w450]
              tunnel: [w450] -> w337
              tunnel: [w449] -> w336
              tunnel: w342 -> [w449]
              tunnel: [w448] -> w335
              tunnel: w341 -> [w448]
              tunnel: w329 -> [w447]
              tunnel: [w447] -> w328
              tunnel: [w446] -> w319
              tunnel: w340 -> [w482]
              tunnel: [w480] -> w362
              tunnel: w339 -> [w479]
              tunnel: w338 -> [w478]
              tunnel: [w478] -> w359
              tunnel: [w477] -> w358
              tunnel: w337 -> [w477]
              tunnel: [w476] -> w357
              tunnel: w336 -> [w476]
              tunnel: w335 -> [w475]
              tunnel: [w474] -> w333
              tunnel: [w473] -> w327
              tunnel: w328 -> [w473]
              tunnel: [w472] -> w320
              tunnel: w319 -> [w472]
              frame #0 {
                n77 = flat-sequence {
                  tunnel: w388 -> [w402]
                  tunnel: [w399] -> w387
                  tunnel: w368 -> [w397]
                  frame #0 {
                    n78 = Reciprocal(x=w402) -> (1/x=w403:dbl)
                    n79 = call <vilib>:"Butterworth Filter PtByPt.vi"("order"=1, "filter type"=Filter_Passband_Type."Lowpass", "low cutoff freq: fl"=20.0, "sampling freq: fs"=w403, "x"=w397) -> ("Filtered x"=w399:dbl)  [unwired: 4 in, 1 out]
                  }
                }
                n80 = call <vilib>:"Read.vi"("AI Ref In"=w382) -> ("Values"=w385:dbl[], "AI Ref Out"=w377:T31)  [unwired: 8 in, 1 out]
                n81 = Divide(x=w389, y=1000000) -> (x/y=w388:dbl)
                n82 = call <vilib>:"Read.vi"("AI Ref In"=w392) -> ("Values"=w391:dbl[], "AI Ref Out"=w376:T31)  [unwired: 8 in, 1 out]
                n83 = Index Array(array=w385, index=0) -> (element=w384:dbl)
                n84 = call <vilib>:"Read.vi"("Encoder Ref In"=w395) -> ("Counter Value"=w394:i32, "Encoder Ref Out"=w378:T29)  [unwired: 6 in, 3 out]
                n85 = call "TF_MotorCurrentInput.vi"("Motor Current Monitor Value [V]"=w384) -> ("Current [A]"=w383:dbl)
                n86 = call "Tacho2Velocity_params.vi"() -> ("Cluster"=w370:T34)  [unwired: 5 in]
                n87 = Index Array(array=w391, index=0) -> (element=w369:dbl)
                n88 = local write "Boolean: Apply Current"(FALSE) -> ()
                n89 = call "TF_Encoder2Position.vi"("Counter Value"=w394, "Offset"=0.0) -> ("Position [deg]"=w373:dbl)  [unwired: 3 in]
                n90 = local write "Boolean: Move"(TRUE) -> ()
                n91 = local write "Position [deg]"(w373) -> ()
                n92 = call "TF_Tacho2Velocity.vi"("Tachometer Voltage [V]"=w369, "Tachometer param"=w370) -> ("Tachometer Velocity [deg/s]"=w368:dbl)  [unwired: 2 in]
                n93 = local write "Current [A] Chart"(w383) -> ()
                "Velocity [deg/s]" <- w387
              }
              frame #1 {
                n94 = First Call?() -> (First Call?: T/F=w429:bool)
                n95 = Or(x=w429, y=w428) -> (x .or. y?=w427:bool)
                n96 = Index Array(array=w412, index=w413) -> (element=w410:dbl)
                n97 = feedback #1() -> (w421:cluster{"time (s)":dbl, "setpoint":dbl}[])  [unwired: 1 in]
                n98 = case shown="True" w427 {
                  tunnel: [w436 w437] -> w420
                  tunnel: w421 -> [w436 _]
                  tunnel: w413 -> [w435 w444]
                  tunnel: w412 -> [_ w445]
                  tunnel: [w435 w443] -> w417
                  tunnel: w414 -> [_ w442]
                  frame False {
                  }
                  frame True {
                    # "Final Position"
                    n99 = Index Array(array=w445, index=w444) -> (element=w441:dbl)
                    n100 = call "motion_create_minimum_jerk.vi"("Initial Position"=w442, "Final Position"=w441, "Initial Time [s]"=0.0, "Final Time [s]"=1.0, "Delta Time [s]"=0.01) -> ("Profile"=w437:cluster{"time (s)":dbl, "setpoint":dbl}[])  [unwired: 10 in]
                    n101 = Increment(x=w444) -> (x+1=w443:dbl)
                  }
                }
                n102 = feedback-in #1(w420) -> ()
                n103 = Greater Or Equal?(x=w410, y=95.0) -> (x >= y?=w416:bool)
                n104 = case shown="True" w416 {
                  tunnel: [FALSE TRUE] -> w415
                  frame False {
                  }
                  frame True {
                    n105 = local write "move"(FALSE) -> ()
                  }
                }
                n106 = call <vilib>:"PID Setpoint Profile.vi"("reinitialize? (F)"=w427, "dt (s)"=w405, "setpoint profile"=w420) -> ("profile complete?"=w419:bool, "setpoint"=w408:dbl)  [unwired: 3 in, 2 out]
                "Profile Complete?" <- w419
                n107 = call "ENPID.vi"("PID Settings"="PID Settings", "r"=w408, "y"=w407, "dy/dt"=w406, "dt (s)"=w405) -> ("u"=w409:dbl)  [unwired: 13 in, 1 out]
                n108 = case shown="False" w419 {
                  tunnel: [w433 0.0] -> w418
                  tunnel: w409 -> [w433 _]
                  frame False {
                  }
                  frame True {
                  }
                }
              }
              frame #2 {
                n109 = call "TF_MotorCurrentOutput.vi"("Motor Current Setpoint [A]"=w455) -> ("Motor Current Setpoint [V]"=w454:dbl)
                n110 = flat-sequence "Safety" {
                  tunnel: w454 -> [w471]
                  tunnel: [w470] -> w453
                  tunnel: w446 -> [w467]
                  frame #0 {
                    w459 = 0.0  # [V]
                    w465 = 0.0  # [V]
                    w468 = 90.0  # [deg]
                    w469 = 90.0  # [deg]
                    w461 = -10.0  # [V]
                    w466 = 10.0  # [V]
                    n111 = In Range and Coerce(upper limit=w466, x=w471, lower limit=w461) -> (coerced(x)=w462:dbl)  [unwired: 1 out]
                    n112 = Less Or Equal?(x=w467, y=w469) -> (x <= y?=w456:bool)
                    n113 = Greater Or Equal?(x=w467, y=w468) -> (x >= y?=w460:bool)
                    n114 = And(x=w456, y=w460) -> (x .and. y?=w457:bool)
                    n115 = Select(t=w466, s=w456, f=w465) -> (s? t:f=w463:dbl)
                    n116 = Select(t=w461, s=w460, f=w459) -> (s? t:f=w458:dbl)
                    n117 = In Range and Coerce(upper limit=w463, x=w462, lower limit=w458) -> (coerced(x)=w464:dbl)  [unwired: 1 out]
                    n118 = Select "Within Position Range?"(t=w462, s=w457, f=w464) -> (s? t:f=w470:dbl)
                  }
                }
              }
              frame #3 {
                # "Motor Current Setpoint"
                n119 = case shown="True" w475 {
                  tunnel: [TypeDef_Static_Friction."Move" ("Actions") TypeDef_Static_Friction."Wait" ("Actions")] -> w474
                  frame False {
                  }
                  frame True {
                  }
                }
                n120 = Build Array(w482) -> (w481:dbl[])
                n121 = call <vilib>:"Write.vi"("Values"=w481, "AO Ref In"=w479) -> ("AO Ref Out"=w480:T21)  [unwired: 7 in, 1 out]
              }
            }
          }
          frame "Wait" {
            n122 = Equal?(x=1000, y=w494) -> (x = y?=w502:bool)
            n123 = local write "Boolean: Apply Current"(FALSE) -> ()
            n124 = Select(t=0, s=w502, f=w494) -> (s? t:f=w500:i32)
            n125 = Increment(x=w500) -> (x+1=w492:i32)
            n126 = case shown="True" w502 {
              tunnel: [TypeDef_Static_Friction."Wait" ("Actions") TypeDef_Static_Friction."Apply Current" ("Actions")] -> w505
              frame False {
              }
              frame True {
              }
            }
            n127 = Build Array(0.0) -> (w508:dbl[])
            n128 = local write "Boolean: Move"(FALSE) -> ()
            n129 = call <vilib>:"Write.vi"("Values"=w508, "AO Ref In"=w504) -> ("AO Ref Out"=w503:T21)  [unwired: 7 in, 1 out]
            n130 = call <vilib>:"Read.vi"("Encoder Ref In"=w488) -> ("Counter Value"=w487:i32, "Encoder Ref Out"=w489:T29)  [unwired: 6 in, 3 out]
            n131 = call "TF_Encoder2Position.vi"("Counter Value"=w487, "Offset"=0.0) -> ("Position [deg]"=w485:dbl)  [unwired: 3 in]
          }
          frame "Apply Current" {
            n132 = flat-sequence {
              tunnel: w531 -> [w584]
              tunnel: w530 -> [w579]
              tunnel: [w571] -> w560
              tunnel: [w576] -> w559
              tunnel: w528 -> [w576]
              tunnel: w526 -> [w573]
              tunnel: [w574] -> w558
              tunnel: w524 -> [w570]
              tunnel: [w571] -> w557
              tunnel: [w570] -> w556
              tunnel: [w569] -> w555
              tunnel: w523 -> [w568]
              tunnel: [w568] -> w554
              tunnel: [w567] -> w553
              tunnel: w522 -> [w567]
              tunnel: [w566] -> w552
              tunnel: [w565] -> w551
              tunnel: w560 -> [w585]
              tunnel: w559 -> [w596]
              tunnel: w558 -> [w600]
              tunnel: w557 -> [w598]
              tunnel: w556 -> [w597]
              tunnel: w555 -> [w589]
              tunnel: [w591] -> w550
              tunnel: [w590] -> w549
              tunnel: [w599] -> w548
              tunnel: [w585] -> w547
              tunnel: [w590] -> w546
              tunnel: w554 -> [w595]
              tunnel: [w595] -> w545
              tunnel: [w594] -> w544
              tunnel: w553 -> [w594]
              tunnel: w552 -> [w593]
              tunnel: [w593] -> w543
              tunnel: [w592] -> w542
              tunnel: w551 -> [w592]
              tunnel: [w585] -> w541
              tunnel: w550 -> [w624]
              tunnel: [w624] -> w540
              tunnel: w549 -> [w629]
              tunnel: [w629] -> w539
              tunnel: w548 -> [w635]
              tunnel: [w635] -> w538
              tunnel: w547 -> [w634]
              tunnel: [w634] -> w537
              tunnel: w546 -> [w628]
              tunnel: [w626] -> w536
              tunnel: w545 -> [w633]
              tunnel: [w633] -> w535
              tunnel: w544 -> [w632]
              tunnel: [w632] -> w534
              tunnel: w543 -> [w631]
              tunnel: [w631] -> w533
              tunnel: w542 -> [w630]
              tunnel: [w630] -> w532
              tunnel: w541 -> [w625]
              tunnel: [w660] -> w525
              tunnel: [w661] -> w527
              tunnel: [w662] -> w529
              tunnel: [w652] -> w516
              tunnel: w540 -> [w652]
              tunnel: w539 -> [w662]
              tunnel: w538 -> [w661]
              tunnel: w537 -> [w660]
              tunnel: w536 -> [w658]
              tunnel: w535 -> [w657]
              tunnel: [w656] -> w520
              tunnel: [w655] -> w521
              tunnel: w534 -> [w655]
              tunnel: w533 -> [w654]
              tunnel: [w654] -> w519
              tunnel: w532 -> [w653]
              tunnel: [w653] -> w518
              frame #0 {
                n133 = call <vilib>:"Read.vi"("AI Ref In"=w584) -> ("Values"=w582:dbl[], "AI Ref Out"=w565:T31)  [unwired: 8 in, 1 out]
                n134 = Equal?(x=1000, y=w573) -> (x = y?=w569:bool)
                n135 = call <vilib>:"Read.vi"("Encoder Ref In"=w579) -> ("Counter Value"=w578:i32, "Encoder Ref Out"=w566:T29)  [unwired: 6 in, 3 out]
                n136 = Index Array(array=w582, index=0) -> (element=w581:dbl)
                n137 = call "TF_Encoder2Position.vi"("Counter Value"=w578, "Offset"=0.0) -> ("Position [deg]"=w571:dbl)  [unwired: 3 in]
                "Position [deg]" <- w571
                "Position [deg] Chart" <- w571
                n138 = Select(t=0, s=w569, f=w573) -> (s? t:f=w574:i32)
                n139 = call "TF_MotorCurrentInput.vi"("Motor Current Monitor Value [V]"=w581) -> ("Current [A]"=→"Current [A]" →"Current [A] Chart":dbl)
                "Boolean: Apply Current" <- TRUE
                "Boolean: Move" <- FALSE
              }
              frame #1 {
                n140 = case shown="\"Positive\", Default" "Current Direction [+/-]" {
                  tunnel: w598 -> [w605 w607]
                  tunnel: w597 -> [w604 w608]
                  tunnel: [w602 w609] -> w591
                  tunnel: [w601 w606] -> w588
                  frame "Positive", Default {
                    n141 = Subtract(x=w605, y=w604) -> (x-y=w601:dbl)
                    n142 = Greater Or Equal?(x=w601, y=0.015) -> (x >= y?=w602:bool)
                  }
                  frame "Negative" {
                    n143 = Subtract(x=w608, y=w607) -> (x-y=w606:dbl)
                    n144 = Greater Or Equal?(x=w606, y=0.015) -> (x >= y?=w609:bool)
                  }
                }
                "Position Difference [deg]" <- w588
                n145 = Increment(x=w600) -> (x+1=w599:i32)
                n146 = case shown="True" w589 {
                  tunnel: w596 -> [w614 w617]
                  tunnel: [w614 w616] -> w587
                  tunnel: "Current Direction [+/-]" -> [_ w615]
                  frame False {
                  }
                  frame True {
                    n147 = case shown="\"Positive\", Default" w615 {
                      tunnel: w617 -> [w619 w622]
                      tunnel: [w618 w621] -> w616
                      frame "Positive", Default {
                        w620 = 0.001  # Current increment [A]
                        n148 = Add(x=w620, y=w619) -> (x+y=w618:dbl)
                      }
                      frame "Negative" {
                        w623 = 0.001  # Current increment [A]
                        n149 = Subtract(x=w622, y=w623) -> (x-y=w621:dbl)
                      }
                    }
                  }
                }
                "Current Setpoint [A]" <- w587
                n150 = case shown="True" w591 {
                  tunnel: [w611 0.0] -> w590
                  tunnel: w587 -> [w611 w612]
                  frame False {
                  }
                  frame True {
                    "Final Current Setpoint" <- w612
                  }
                }
              }
              frame #2 {
                n151 = flat-sequence "Safety" {
                  tunnel: w627 -> [w651]
                  tunnel: [w650] -> w626
                  tunnel: w625 -> [w647]
                  frame #0 {
                    w639 = 0.0  # [V]
                    w645 = 0.0  # [V]
                    w648 = -85.0  # [deg]
                    w649 = 85.0  # [deg]
                    w641 = -10.0  # [V]
                    w646 = 10.0  # [V]
                    n152 = In Range and Coerce(upper limit=w646, x=w651, lower limit=w641) -> (coerced(x)=w642:dbl)  [unwired: 1 out]
                    n153 = Less Or Equal?(x=w647, y=w649) -> (x <= y?=w636:bool)
                    n154 = Greater Or Equal?(x=w647, y=w648) -> (x >= y?=w640:bool)
                    n155 = And(x=w636, y=w640) -> (x .and. y?=w637:bool)
                    n156 = Select(t=w646, s=w636, f=w645) -> (s? t:f=w643:dbl)
                    n157 = Select(t=w641, s=w640, f=w639) -> (s? t:f=w638:dbl)
                    n158 = In Range and Coerce(upper limit=w643, x=w642, lower limit=w638) -> (coerced(x)=w644:dbl)  [unwired: 1 out]
                    n159 = Select "Within Position Range?"(t=w642, s=w637, f=w644) -> (s? t:f=w650:dbl)
                  }
                }
                n160 = call "TF_MotorCurrentOutput.vi"("Motor Current Setpoint [A]"=w628) -> ("Motor Current Setpoint [V]"=w627:dbl)
              }
              frame #3 {
                # "Motor Current Setpoint"
                n161 = Build Array(w658) -> (w659:dbl[])
                n162 = call <vilib>:"Write.vi"("Values"=w659, "AO Ref In"=w657) -> ("AO Ref Out"=w656:T21)  [unwired: 7 in, 1 out]
              }
            }
            n163 = case shown="True" w516 {
              tunnel: [TypeDef_Static_Friction."Apply Current" ("Actions") TypeDef_Static_Friction."Move" ("Actions")] -> w515
              frame False {
              }
              frame True {
              }
            }
          }
        }
        n164 = Or(x="stop", y=w268) -> (x .or. y?=w269:bool)
        n165 = case shown="True" "stop" {
          frame False {
          }
          frame True {
            n166 = local write "move"(FALSE) -> ()
          }
        }
        n167 = node-c288() -> ()  [unwired: 1 in, 1 out]
      }
      n168 = node-c288(w155) -> ()  [unwired: 1 out]
      n169 = node-c288(w175) -> ()  [unwired: 1 out]
    }
    frame #5 {
      # "Tachometer"
      # "Motor Current Monitor"
      # "Motor Current Setpoint"
      # "Encoder"
      # "Reset"
      # "Close Everything"
      n170 = call <vilib>:"Close.vi"("AI Ref In"=w671) -> ()  [unwired: 10 in, 1 out]
      n171 = Build Array(0.0) -> (w674:dbl[])
      n172 = call <vilib>:"Close.vi"("AI Ref In"=w670) -> ()  [unwired: 10 in, 1 out]
      n173 = call <vilib>:"Stop.vi"("Encoder Ref In"=w672) -> ("Encoder Ref Out"=w677:T29)  [unwired: 9 in, 1 out]
      n174 = call <vilib>:"Close.vi"("AO Ref In"=w678) -> ()  [unwired: 10 in, 1 out]
      n175 = call <vilib>:"Write.vi"("Values"=w674, "AO Ref In"=w673) -> ("AO Ref Out"=w676:T21)  [unwired: 7 in, 1 out]
      n176 = call <vilib>:"Close.vi"("Encoder Ref In"=w677) -> ()  [unwired: 10 in, 1 out]
      n177 = call <vilib>:"Close.vi"("AO Ref In"=w676) -> ()  [unwired: 10 in, 1 out]
    }
  }
